vi "Brain.vi"(8 "Index":T1={"N1"=18, "N2"=19, "N3"=4, "N4"=5, "V1"=8, "V2"=10, "V3"=10, "V4"=13, "CURRENT"=12, "Vsg"=1}, 9 "voltage":bool=TRUE, 10 "Conductance In":T2(graph), 11 "Folder Path":path) -> (2 "Conductance Out":T2(graph))   [LabVIEW 2016]
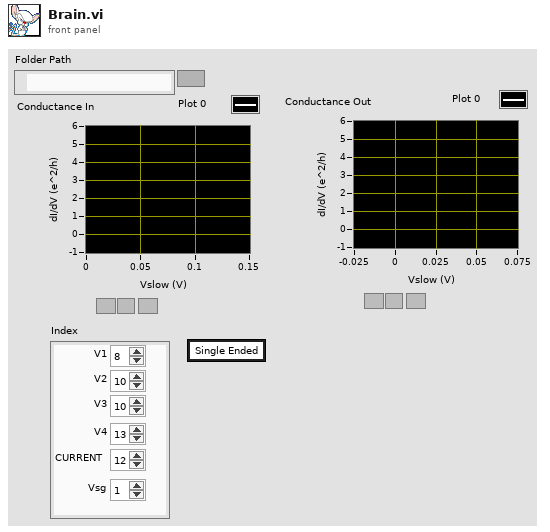
[diagram p1: front panel]
types:
  T1 = cluster{"N1":i32, "N2":i32, "N3":i32, "N4":i32, "V1":i32, "V2":i32, "V3":i32, "V4":i32, "CURRENT":i32, "Vsg":i32}
  T2 = cluster{"Vfast":dbl[], "Decimated Array":dbl[]}[]
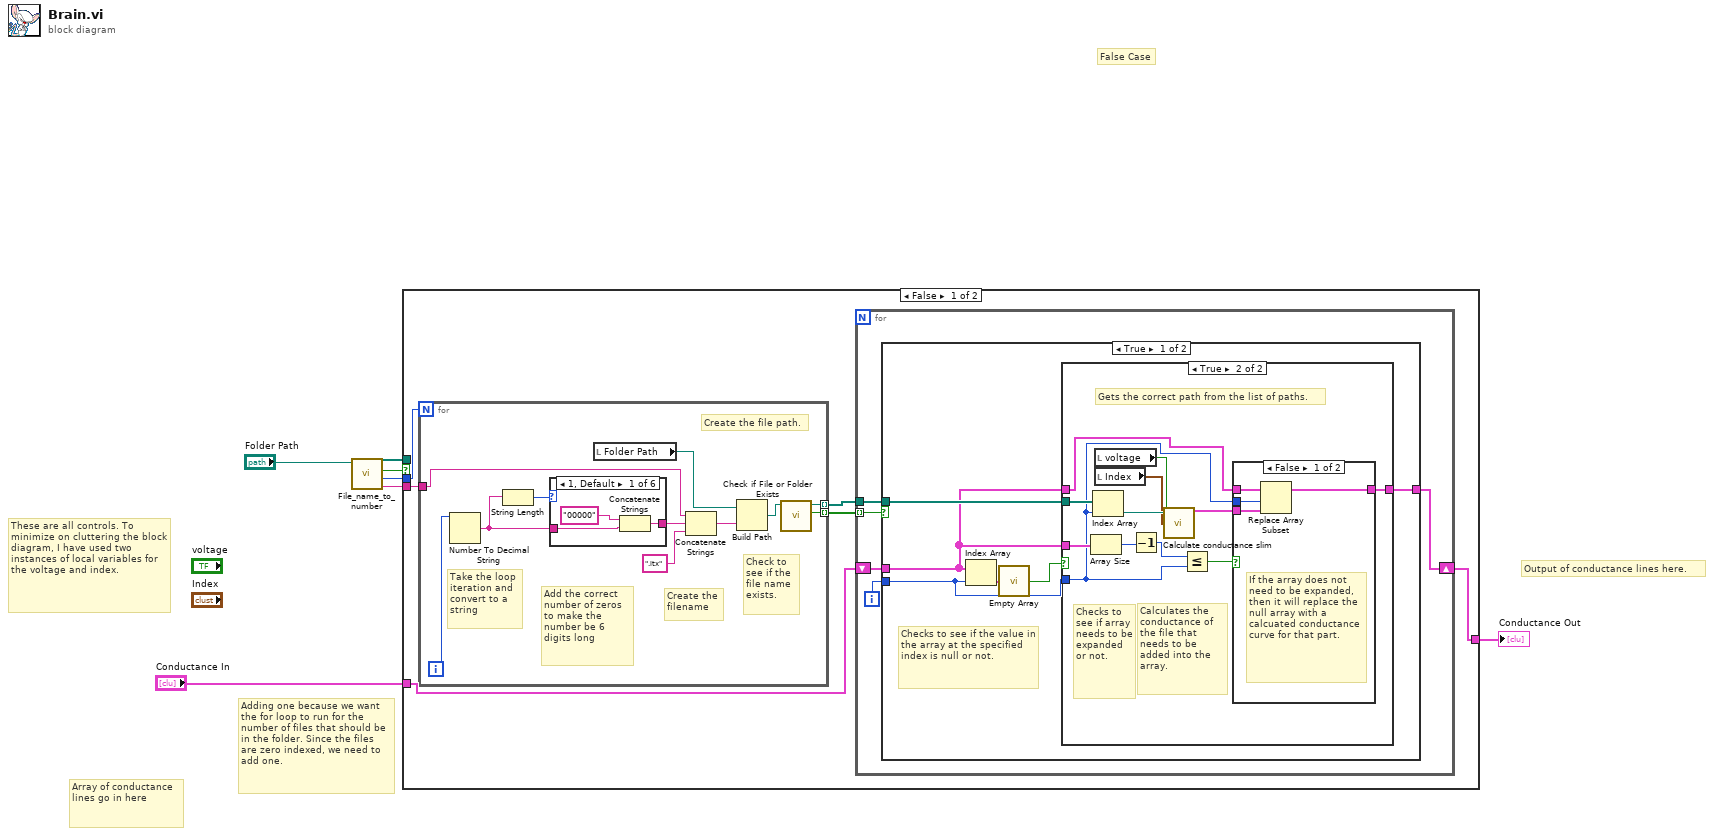
[diagram p0: block diagram]
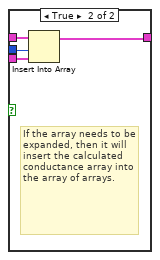
[diagram p3: hidden frame]
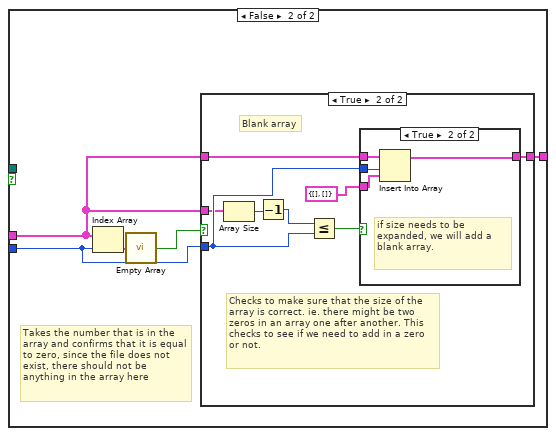
[diagram p4: hidden frame]
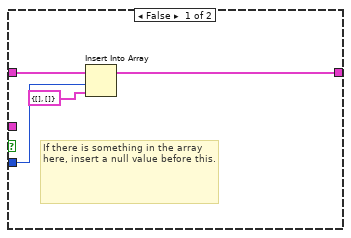
[diagram p5: hidden frame]
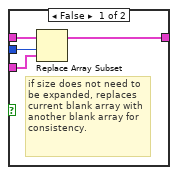
[diagram p6: hidden frame]
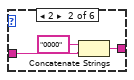
[diagram p7: hidden frame]
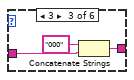
[diagram p8: hidden frame]
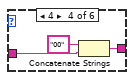
[diagram p9: hidden frame]
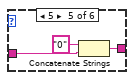
[diagram p10: hidden frame]
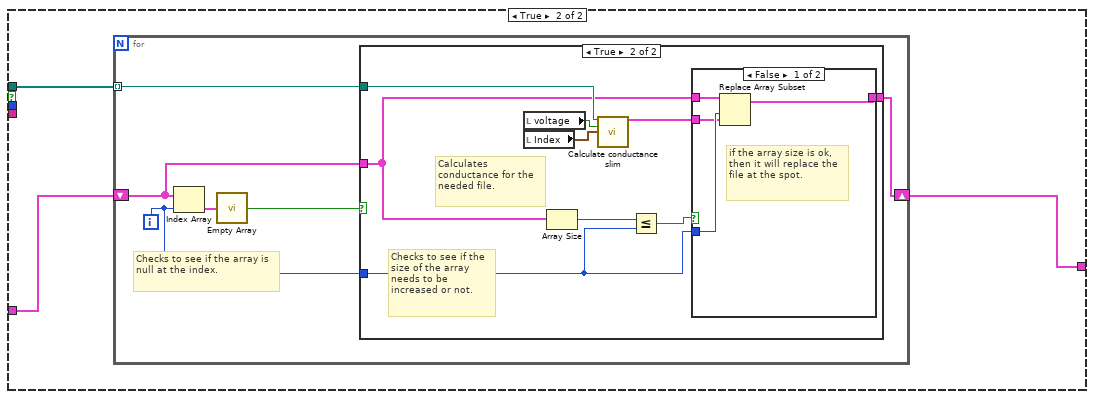
[diagram p12: hidden frame]
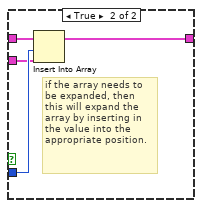
[diagram p14: hidden frame]
diagram:
  # "Output of conductance lines here."
  # "Array of conductance lines go in here"
  # "Adding one because we want the for loop to run for the number of files that should be in the folder. Since the files are zero indexed, we need to add one."
  # "False Case"
  # "These are all controls. To minimize on cluttering the block diagram, I have used two instances of local variables for the voltage and index."
  n1 = call "File_name_to_number.vi"("Folder Path"="Folder Path") -> ("Base File Name"=w1:string, "Last file number"=w5:i32, "File number =  file name?"=w6:bool, "All Files in Dir"=w3:path[])  [unwired: 6 in]
  n2 = case shown="False" w6 {
    tunnel: w5 -> [w13 _]
    tunnel: w1 -> [w12 _]
    tunnel: "Conductance In" -> [w9 w100]
    tunnel: [w8 w98] -> w2
    tunnel: w3 -> [_ w99]
    frame False {
      n3 = for {
        N: w13 -> [_]
        tunnel: w12 -> [w78]
        tunnel: [w72] -> w11 mode=indexing
        tunnel: [w71] -> w10 mode=indexing
        i -> [w81]
        # "Check to see if the file name exists."
        # "Create the file path."
        # "Create the filename"
        # "Add the correct number of zeros to make the number be 6 digits long"
        # "Take the loop iteration and convert to a string"
        n4 = Number To Decimal String(number=w81) -> (decimal integer string=w79:string)  [unwired: 1 in]
        n5 = String Length(string=w79) -> (length=w80:i32)
        n6 = case shown="1, Default" w80 {
          tunnel: w79 -> [w84 w87 w90 w93 w96 w97]
          tunnel: [w82 w86 w89 w92 w95 w97] -> w77
          frame 1, Default {
            n7 = Concatenate Strings("00000" ("string"), w84) -> (w82:string)
          }
          frame 2 {
            n8 = Concatenate Strings("0000" ("string"), w87) -> (w86:string)
          }
          frame 3 {
            n9 = Concatenate Strings("000" ("string"), w90) -> (w89:string)
          }
          frame 4 {
            n10 = Concatenate Strings("00" ("string"), w93) -> (w92:string)
          }
          frame 5 {
            n11 = Concatenate Strings("0" ("string"), w96) -> (w95:string)
          }
          frame 6 {
          }
        }
        n12 = local read "Folder Path"() -> (w74:path)
        n13 = Concatenate Strings(w78, w77, ".itx" ("string")) -> (w75:string)
        n14 = Build Path(base path=w74, name or relative path=w75) -> (appended path=w73:path)
        n15 = call <vilib>:"Check if File or Folder Exists.vi"("path"=w73) -> ("file or folder exists?"=w72:bool, "dup path"=w71:path)  [unwired: 8 in, 1 out]
      }
      n16 = for {
        tunnel: w11 -> [w18] mode=indexing
        tunnel: w10 -> [w15]
        shift-right: [w14] -> w8
        shift-left: w9 -> [w17]
        i -> [w16]
        n17 = case shown="True" w18 {
          tunnel: w17 -> [w20 w46]
          tunnel: w16 -> [w22 w48]
          tunnel: w15 -> [w21 _]
          tunnel: [w19 w47] -> w14
          frame True {
            # "Checks to see if the value in the array at the specified index is null or not."
            n18 = Index Array(array=w20, index=w22) -> (element=w24:cluster{"Vfast":dbl[], "Decimated Array":dbl[]})
            n19 = call "Empty Array.vi"("Cluster"=w24) -> ("Boolean"=w23:bool)  [unwired: 8 in]
            n20 = case shown="True" w23 {
              tunnel: w20 -> [_ w34]
              tunnel: w22 -> [_ w27]
              tunnel: w21 -> [_ w35]
              tunnel: w20 -> [w25 w26]
              tunnel: [w25 w30] -> w19
              frame False {
                # "If the value is not null, it leaves it alone. This prevents the program from having to calculate the conductance of every file in the folder every time something is added to it."
              }
              frame True {
                # "Gets the correct path from the list of paths."
                # "Calculates the conductance of the file that needs to be added into the array."
                # "Checks to see if array needs to be expanded or not."
                n21 = Array Size(array=w34) -> (size(s)=w37:i32)
                n22 = Index Array(array=w35, index=w27) -> (element=w33:path)
                n23 = local read "voltage"() -> (w29:bool)
                n24 = local read "Index"() -> (w28:T1)
                n25 = Decrement(x=w37) -> (x-1=w36:i32)
                n26 = call "Calculate conductance slim.vi"("File or Folder Path"=w33, "single ended?"=w29, "index"=w28) -> ("A vs D"=w31:cluster{dbl[], dbl[]}[])  [unwired: 12 in]
                n27 = Less Or Equal?(x=w36, y=w27) -> (x <= y?=w32:bool)
                n28 = case shown="False" w32 {
                  tunnel: w31 -> [w41 w44]
                  tunnel: w26 -> [w40 w45]
                  tunnel: w27 -> [w39 w43]
                  tunnel: [w38 w42] -> w30
                  frame False {
                    # "If the array does not need to be expanded, then it will replace the null array with a calcuated conductance curve for that part."
                    n29 = Replace Array Subset(array=w40, new element=w41, index=w39) -> (w38:T2)
                  }
                  frame True {
                    # "If the array needs to be expanded, then it will insert the calculated conductance array into the array of arrays."
                    n30 = Insert Into Array(array=w45, index=w43, new element=w44) -> (w42:T2)
                  }
                }
              }
            }
          }
          frame False {
            # "Takes the number that is in the array and confirms that it is equal to zero, since the file does not exist, there should not be anything in the array here"
            n31 = Index Array(array=w46, index=w48) -> (element=w50:cluster{"Vfast":dbl[], "Decimated Array":dbl[]})
            n32 = call "Empty Array.vi"("Cluster"=w50) -> ("Boolean"=w49:bool)  [unwired: 8 in]
            n33 = case shown="True" w49 {
              tunnel: w48 -> [w52 w58]
              tunnel: w46 -> [w54 w59]
              tunnel: [w53 w57] -> w47
              tunnel: w46 -> [_ w56]
              frame False {
                # "If there is something in the array here, insert a null value before this."
                n34 = Insert Into Array(array=w54, index=w52, new element=cluster{"Vfast":dbl[], "Decimated Array":dbl[]} {"Vfast"=[], "Decimated Array"=[]} ("x")) -> (w53:T2)
              }
              frame True {
                # "Blank array"
                # "Checks to make sure that the size of the array is correct. ie. there might be two zeros in an array one after another. This checks to see if we need to add in a zero or not."
                n35 = Array Size(array=w56) -> (size(s)=w62:i32)
                n36 = Decrement(x=w62) -> (x-1=w61:i32)
                n37 = Less Or Equal?(x=w61, y=w58) -> (x <= y?=w60:bool)
                n38 = case shown="True" w60 {
                  tunnel: w59 -> [w66 w70]
                  tunnel: w58 -> [w65 w69]
                  tunnel: [w64 w68] -> w57
                  tunnel: cluster{"Vfast":dbl[], "Decimated Array":dbl[]} {"Vfast"=[], "Decimated Array"=[]} ("x") -> [w63 w67]
                  frame False {
                    # "if size does not need to be expanded, replaces current blank array with another blank array for consistency."
                    n39 = Replace Array Subset(array=w66, new element=w63, index=w65) -> (w64:T2)
                  }
                  frame True {
                    # "if size needs to be expanded, we will add a blank array."
                    n40 = Insert Into Array(array=w70, index=w69, new element=w67) -> (w68:T2)
                  }
                }
              }
            }
          }
        }
      }
    }
    frame True {
      n41 = for {
        shift-right: [w102] -> w98
        shift-left: w100 -> [w103]
        tunnel: w99 -> [w104] mode=indexing
        i -> [w101]
        # "Checks to see if the array is null at the index."
        n42 = Index Array(array=w103, index=w101) -> (element=w106:cluster{"Vfast":dbl[], "Decimated Array":dbl[]})
        n43 = call "Empty Array.vi"("Cluster"=w106) -> ("Boolean"=w105:bool)  [unwired: 8 in]
        n44 = case shown="True" w105 {
          tunnel: w104 -> [_ w110]
          tunnel: w103 -> [w107 w108]
          tunnel: [w107 w113] -> w102
          tunnel: w101 -> [_ w109]
          frame False {
            # "if the value is not null, then it will ignore the value."
          }
          frame True {
            # "Calculates conductance for the needed file."
            # "Checks to see if the size of the array needs to be increased or not."
            n45 = local read "voltage"() -> (w112:bool)
            n46 = local read "Index"() -> (w111:T1)
            n47 = Array Size(array=w108) -> (size(s)=w116:i32)
            n48 = call "Calculate conductance slim.vi"("File or Folder Path"=w110, "single ended?"=w112, "index"=w111) -> ("A vs D"=w114:cluster{dbl[], dbl[]}[])  [unwired: 12 in]
            n49 = Less Or Equal?(x=w116, y=w109) -> (x <= y?=w115:bool)
            n50 = case shown="False" w115 {
              tunnel: w108 -> [w120 w124]
              tunnel: w109 -> [w119 w123]
              tunnel: w114 -> [w118 w122]
              tunnel: [w117 w121] -> w113
              frame False {
                # "if the array size is ok, then it will replace the file at the spot."
                n51 = Replace Array Subset(array=w120, new element=w118, index=w119) -> (w117:T2)
              }
              frame True {
                # "if the array needs to be expanded, then this will expand the array by inserting in the value into the appropriate position."
                n52 = Insert Into Array(array=w124, index=w123, new element=w122) -> (w121:T2)
              }
            }
          }
        }
      }
    }
  }
  "Conductance Out" <- w2
